vi "begin && filter.vi"() -> ()   [LabVIEW 2012, in "LightPipes.lvlib"]
uses:
  LightPipes.lvlib
panel:
  out "field out":T1
  in  "c2":string
  in  "c1":string
  in  "path for pgm file input":string="C:\\Program Files (x86)\\National Instruments\\LabVIEW 2012\\user.lib\\LightPipes\\images\\out.pgm"
  in  "size grid":dbl=0.01
  in  "lambda":dbl=1e-06
  in  "field":T2
  in  "n_grid":u32=256
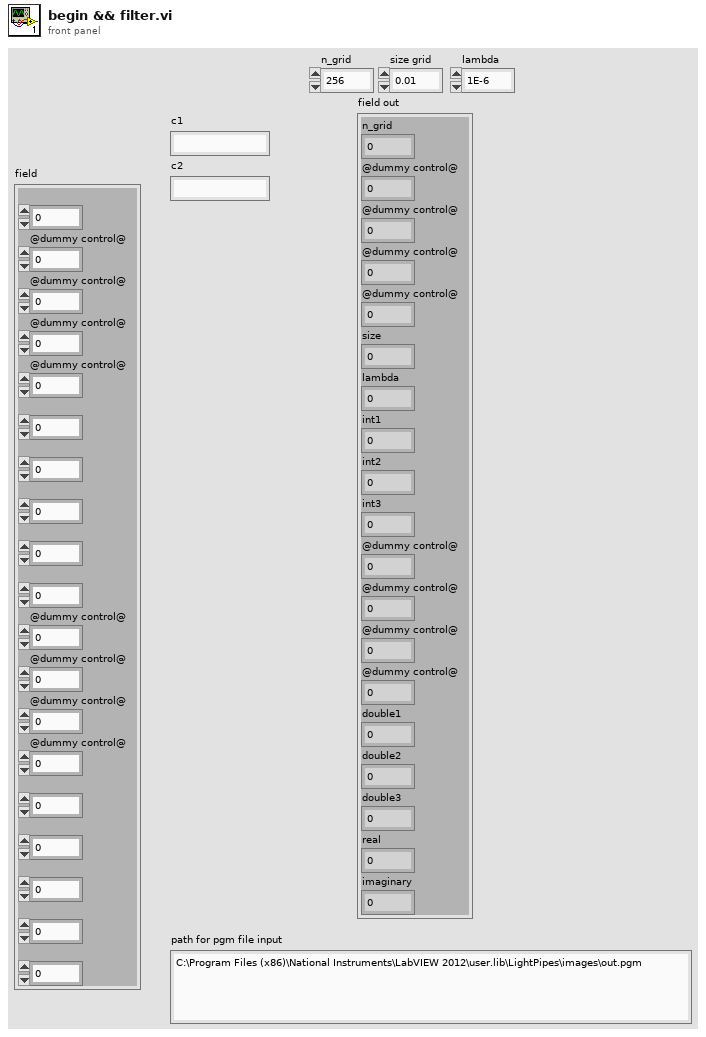
[diagram p1: front panel]
types:
  T1 = cluster{"n_grid":i32, "@dummy control@":i8, "@dummy control@":i8, "@dummy control@":i8, "@dummy control@":i8, "size":dbl, "lambda":dbl, "int1":i32, "int2":i32, "int3":i32, "@dummy control@":i8, "@dummy control@":i8, "@dummy control@":i8, "@dummy control@":i8, "double1":dbl, "double2":dbl, "double3":dbl, "real":u32, "imaginary":u32}
  T2 = cluster{i32, "@dummy control@":i8, "@dummy control@":i8, "@dummy control@":i8, "@dummy control@":i8, dbl, dbl, i32, i32, i32, "@dummy control@":i8, "@dummy control@":i8, "@dummy control@":i8, "@dummy control@":i8, dbl, dbl, dbl, dbl, dbl}
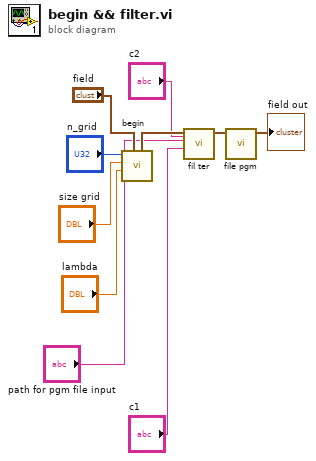
[diagram p0: block diagram]
diagram:
  n1 = call "begin.vi"("field"="field", "lambda"="lambda", "size_grid"="size grid", "n_grid"="n_grid") -> ("field out"=w7:T1)  [unwired: 7 in]
  n2 = call "fil ter.vi"(7:"c2", "multiplication/ substitution"="c1", "intensity / phase"="path for pgm file input", "field"=w7) -> ("field out"=w3:T1)  [unwired: 6 in, 1 out]
  n3 = call "file pgm.vi"("field"=w3) -> ("field out"=→"field out":T1)  [unwired: 9 in, 1 out]
